vi "FPGA_Main.vi"() -> ()   [LabVIEW 2014]
uses:
  Custom Controls/ActuationControl.ctl
  <vilib>/rvi/Emulation/niFpgaGetClockAttributes.vi
  <vilib>/rvi/Emulation/niFpgaSctlEmulationGetInTimedLoop.vi
  <vilib>/rvi/Emulation/niFpgaEmulationReportErrorSimple.vi
  <vilib>/rvi/Emulation/niFpgaProcessEmulError.vi
  <vilib>/rvi/eio/common/nirviEmuTemplateMethod_errors.vi
  <vilib>/rvi/interface/RandomDataEmulation/niFpgaRandomDataHandleErrors.vi
  <vilib>/rvi/Emulation/niFpgaCriticalErrorInLSC.vi
  <vilib>/eio/EIONode/EIONode.xnode
  <vilib>/rvi/DataTransferAndStorage/Container/XNode/niFpgaContainer.xnode
  <vilib>/rvi/interface/RandomDataEmulation/nirviRandomDataFpgaReadWriteTemplate.vi
  <vilib>/rvi/Analysis/measure/butterworth/XNode/niFpgaButterworthFilter.xnode
panel:
  in  "High Pass?":bool
  in  "Low Pass?":bool
  out "ConnectorB/AO0":u16
  in  "Cluster":T1={"Mode"=enum."Stochastic", "Frequency (Periods/tick)"=0.0024999999441206455, "Phase (period)"=0.0}
  in  "Actuation Period (muS)":u32=5
  out "ConnectorB/AI0":u16
  out "Acquistion Timed Out?":bool
  in  "Acquisition Period (muS)":u32=2
  in  "stop":bool
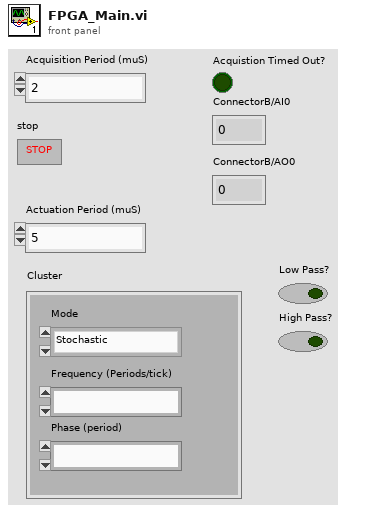
[diagram p1: front panel]
types:
  T1 = typedef "ActuationControl.ctl" = cluster{"Mode":enum16{"Square Wave", "Sine Wave", "White Noise", "Stochastic"}, "Frequency (Periods/tick)":fxp<+,32,0>, "Phase (period)":fxp<+,32,0>}
  T2 = enum16{"Square Wave", "Sine Wave", "White Noise", "Stochastic"}
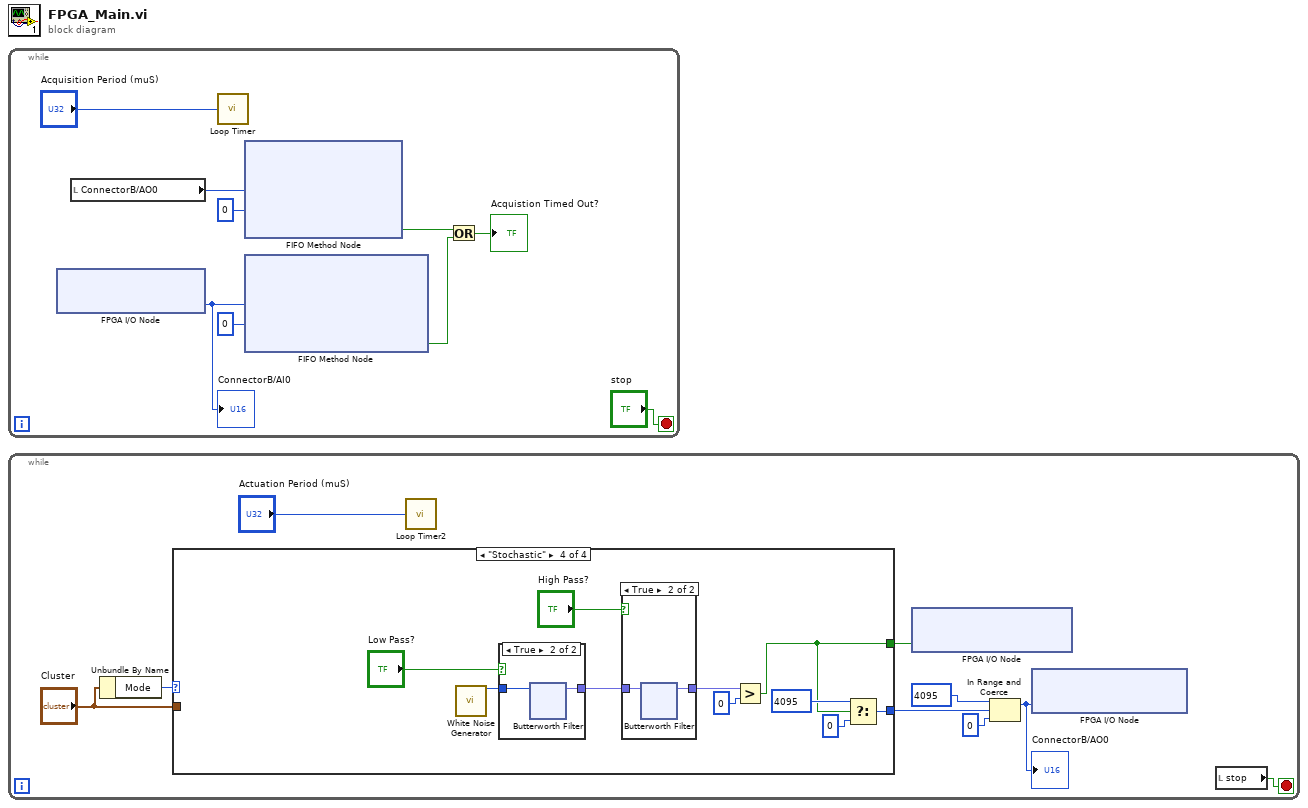
[diagram p0: block diagram]
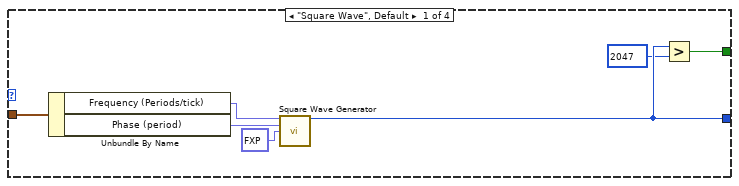
[diagram p2: hidden frame]
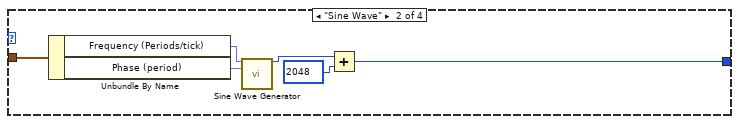
[diagram p3: hidden frame]
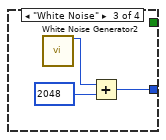
[diagram p4: hidden frame]
diagram:
  n1 = while {
    stop <- "stop" stop-if-true
    n2 = xnode "FPGA I/O Node"() -> ("ConnectorB/AI0"=w8:u16)  [unwired: 1 in, 1 out]
    "ConnectorB/AI0" <- w8
    n3 = local read "ConnectorB/AO0"() -> (w5:u16)
    n4 = call "Loop Timer"("Count(uSec)"="Acquisition Period (muS)") -> ()  [unwired: 1 out]
    n5 = xnode ("FIFO Method Node")("Element"=w5, "Timeout"=0) -> ("Timed Out?"=w2:bool)  [unwired: 1 in, 1 out]
    n6 = xnode ("FIFO Method Node")("Element"=w8, "Timeout"=0) -> ("Timed Out?"=w3:bool)  [unwired: 1 in, 1 out]
    n7 = Or(x=w2, y=w3) -> (x .or. y?=→"Acquistion Timed Out?":bool)
  }
  n8 = while {
    stop <- w17 stop-if-true
    n9 = Unbundle By Name("Cluster") -> ("Mode"=w16:T2)
    n10 = case shown="\"Stochastic\"" w16 {
      tunnel: "Cluster" -> [w25 w28 _ _]
      tunnel: [w21 w30 w32 w41] -> w11
      tunnel: [w19 _ _ w40] -> w10
      frame "Square Wave", Default {
        n11 = Unbundle By Name(w25) -> ("Frequency (Periods/tick)"=w24:fxp<+,32,0>, "Phase (period)"=w23:fxp<+,32,0>)
        n12 = call "Square Wave Generator"("frequency (periods/tick)"=w24, "phase offset (periods)"=w23, "duty cycle (periods)"=fxp<+,32,0> 0.5) -> ("square wave out"=w21:i16)  [unwired: 12 in]
        n13 = Greater?(x=w21, y=i16 2047) -> (0:w19:bool)
      }
      frame "Sine Wave" {
        n14 = Unbundle By Name(w28) -> ("Frequency (Periods/tick)"=w27:fxp<+,32,0>, "Phase (period)"=w26:fxp<+,32,0>)
        n15 = call "Sine Wave Generator"("frequency (periods/tick)"=w27, "phase offset (periods)"=w26) -> ("sine out"=w31:i16)  [unwired: 13 in]
        n16 = Add(x=w31, y=i16 2048) -> (x+y=w30:i16)
      }
      frame "White Noise" {
        n17 = call "White Noise Generator2"() -> ("white noise out"=w33:i16)  [unwired: 15 in]
        n18 = Add(x=w33, y=i16 2048) -> (x+y=w32:i16)
      }
      frame "Stochastic" {
        n19 = call "White Noise Generator"() -> ("white noise out"=w38:i16)  [unwired: 15 in]
        n20 = case shown="True" "Low Pass?" {
          tunnel: w38 -> [w55 w57]
          tunnel: [w55 w56] -> w36
          frame False {
          }
          frame True {
            n21 = xnode "Butterworth Filter"("input data"=w57) -> ("output data"=w56:fxp<+/-,20,20>)  [unwired: 2 in]
          }
        }
        n22 = case shown="True" "High Pass?" {
          tunnel: w36 -> [w45 w47]
          tunnel: [w45 w46] -> w35
          frame False {
          }
          frame True {
            n23 = xnode "Butterworth Filter"("input data"=w47) -> ("output data"=w46:fxp<+/-,24,24>)  [unwired: 2 in]
          }
        }
        n24 = Greater?(x=w35, y=i16 0) -> (0:w40:bool)
        n25 = Select(t=u16 4095 ("y"), s=w40, f=u16 0 ("lower limit")) -> (s? t:f=w41:u16)
      }
    }
    n26 = call "Loop Timer2"("Count(uSec)"="Actuation Period (muS)") -> ()  [unwired: 1 out]
    n27 = xnode "FPGA I/O Node"("ConnectorB/DIO0"=w10) -> ()  [unwired: 1 in, 1 out]
    n28 = In Range and Coerce(upper limit=u16 4095 ("y"), x=w11, lower limit=u16 0) -> (coerced(x)=w12:u16)  [unwired: 1 out]
    "ConnectorB/AO0" <- w12
    n29 = xnode "FPGA I/O Node"("ConnectorB/AO0"=w12) -> ()  [unwired: 1 in, 1 out]
    n30 = local read "stop"() -> (w17:bool)
  }
